vi "Execute.vi"(8 "error in":errorcluster, 11 "Get Max Orifice Flow in":refnum<class "Get Max Orifice Flow.lvclass">) -> (0 "error out":errorcluster, 1 "Next Step?":bool, 2 "MSG":string, 3 "Get Max Orifice Flow out":refnum<class "Get Max Orifice Flow.lvclass">)   [LabVIEW 2015, in "Get Max Orifice Flow.lvclass"]
uses:
  Get Max Orifice Flow.lvclass
  Reusable/Sequence/STEPS/STEP.lvclass/STEP.ctl
  Get Max Orifice Flow.lvclass/Get Max Orifice Flow.ctl
  Controls/MFC Address.ctl
  Reusable/Sequence/STEPS/Read First Call.vi
  Read Max Qorf DVR.vi
  Read WaitTime.vi
  Reusable/Sequence/STEPS/Write First Call.vi
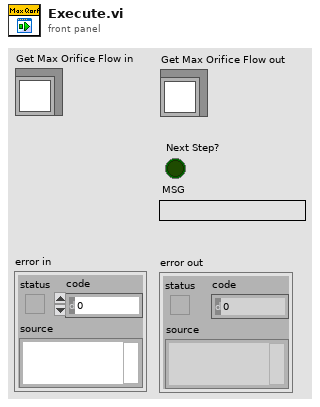
[diagram p1: front panel]
types:
  T1 = typedef "MFC Address.ctl" = enum16{"CRDS Purge", "CRDS Thermodenuded", "CRDS Dry", "CRDS Med RH", "CRDS High RH", "PAS Ch 1", "PAS Ch 2", "PAS Ch3", "PAS Ch 4", "PAS Ch 5", "CLAP", "O3", "Pinlet"}
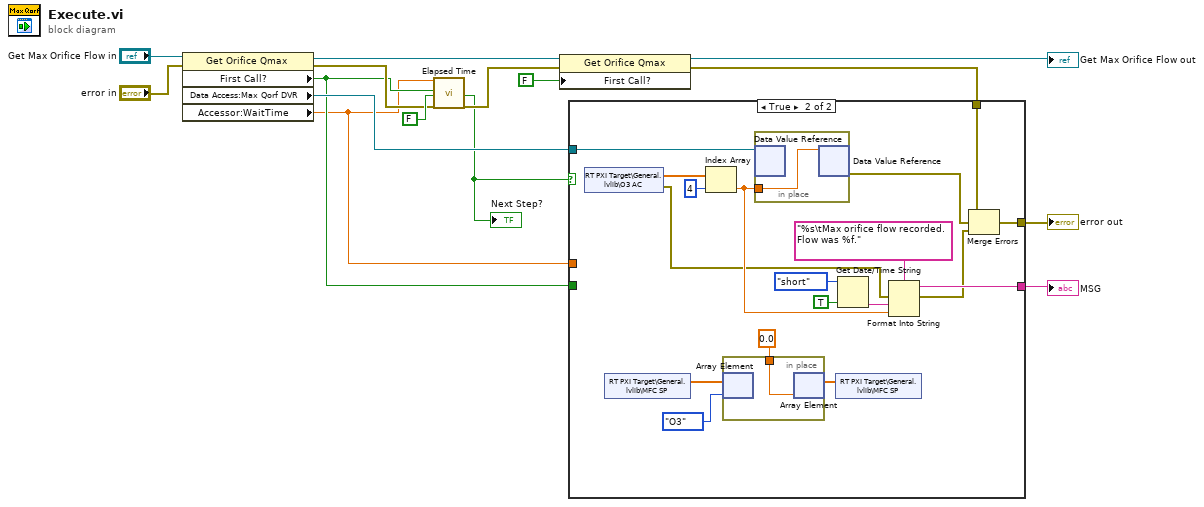
[diagram p0: block diagram]
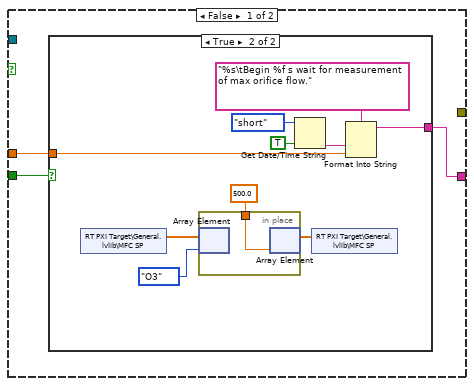
[diagram p2: hidden frame]
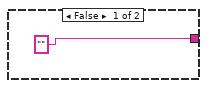
[diagram p3: hidden frame]
diagram:
  n1 = property class="Get Orifice Qmax"(reference="Get Max Orifice Flow in", error in="error in") -> (reference out=w15:refnum<class "Get Max Orifice Flow.lvclass">, error out=w12:errorcluster, "First Call?"=w2:bool, "Data Access:Max Qorf DVR"=w8:refnum<data-value>, "Accessor:WaitTime"=w1:dbl)
  n2 = call "Elapsed Time"("Time Target (s)"=w1, "Reset"=w2, "Auto Reset"=FALSE, "error in (no error)"=w12) -> ("Time has Elapsed"=w6:bool, "error out"=w11:errorcluster)  [unwired: 8 in, 6 out]
  "Next Step?" <- w6
  n3 = property class="Get Orifice Qmax"(reference=w15, error in=w11, "First Call?"=FALSE) -> (reference out=→"Get Max Orifice Flow out":refnum<class "Get Max Orifice Flow.lvclass">, error out=w4:errorcluster)
  n4 = case shown="True" w6 {
    tunnel: w8 -> [_ w48]
    tunnel: [w16 w39] -> w5
    tunnel: [_ w36] -> w3
    tunnel: w4 -> [_ w35]
    tunnel: w2 -> [w18 _]
    tunnel: w1 -> [w17 _]
    frame False {
      n5 = case shown="True" w18 {
        tunnel: w17 -> [_ w25]
        tunnel: ["" w24] -> w16
        frame False {
        }
        frame True {
          n6 = shared-variable "RT PXI Target\\General.lvlib\\MFC SP"() -> (w23:sgl[])  [unwired: 1 in, 1 out]
          n7 = in-place {
            in-place-border: sgl 500.0 ("O2 Flow") -> [w30]
            n8 = in-place-array #1(w23, MFC_Address."O3" ("Controllers")) -> ()  [unwired: 1 out]
            n9 = in-place-array #1(w30) -> (w22:sgl[])  [unwired: 1 out]
          }
          n10 = Get Date/Time String(date format (0)=enum16{"short", "long", "abbreviated"}."short", want seconds? (F)=TRUE) -> (time string=w26:string)  [unwired: 1 in, 1 out]
          n11 = shared-variable "RT PXI Target\\General.lvlib\\MFC SP"(w22) -> ()  [unwired: 1 in, 1 out]
          n12 = Format Into String(format string="%s\tBegin %f s wait for measurement of max orifice flow.", w26, w25) -> (resulting string=w24:string)  [unwired: 2 in, 1 out]
        }
      }
    }
    frame True {
      n13 = shared-variable "RT PXI Target\\General.lvlib\\O3 AC"() -> (w47:sgl[], error out=w40:errorcluster)  [unwired: 1 in]
      n14 = shared-variable "RT PXI Target\\General.lvlib\\MFC SP"() -> (w34:sgl[])  [unwired: 1 in, 1 out]
      n15 = Index Array(array=w47, index=4) -> (element=w41:sgl)
      n16 = in-place {
        in-place-border: sgl 0.0 ("O2 Flow") -> [w49]
        n17 = in-place-array #2(w34, MFC_Address."O3" ("Controllers")) -> ()  [unwired: 1 out]
        n18 = in-place-array #2(w49) -> (w33:sgl[])  [unwired: 1 out]
      }
      n19 = in-place {
        in-place-border: w41 -> [w50]
        n20 = in-place-dvr #3(w48) -> ()  [unwired: 2 out]
        n21 = in-place-dvr #3(w50) -> (w38:errorcluster)  [unwired: 1 out]
      }
      n22 = shared-variable "RT PXI Target\\General.lvlib\\MFC SP"(w33) -> ()  [unwired: 1 in, 1 out]
      n23 = Get Date/Time String(date format (0)=enum16{"short", "long", "abbreviated"}."short", want seconds? (F)=TRUE) -> (time string=w42:string)  [unwired: 1 in, 1 out]
      n24 = Format Into String(format string="%s\tMax orifice flow recorded.   Flow was %f.", error in=w40, w42, w41) -> (resulting string=w39:string, error out=w37:errorcluster)  [unwired: 1 in]
      n25 = Merge Errors(w35, w38, w37) -> (w36:errorcluster)
    }
  }
  "error out" <- w3
  "MSG" <- w5
